vi "Untrained app.vi"() -> ()   [LabVIEW 2024]
panel:
  out "Instrument identificat":string
  in  "Classify":bool
  in  "Cale fisier audio":path
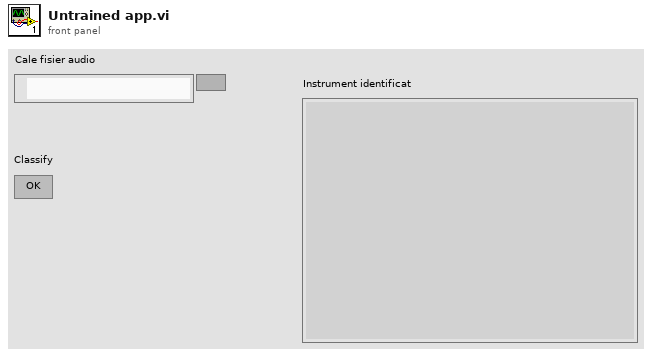
[diagram p1: front panel]
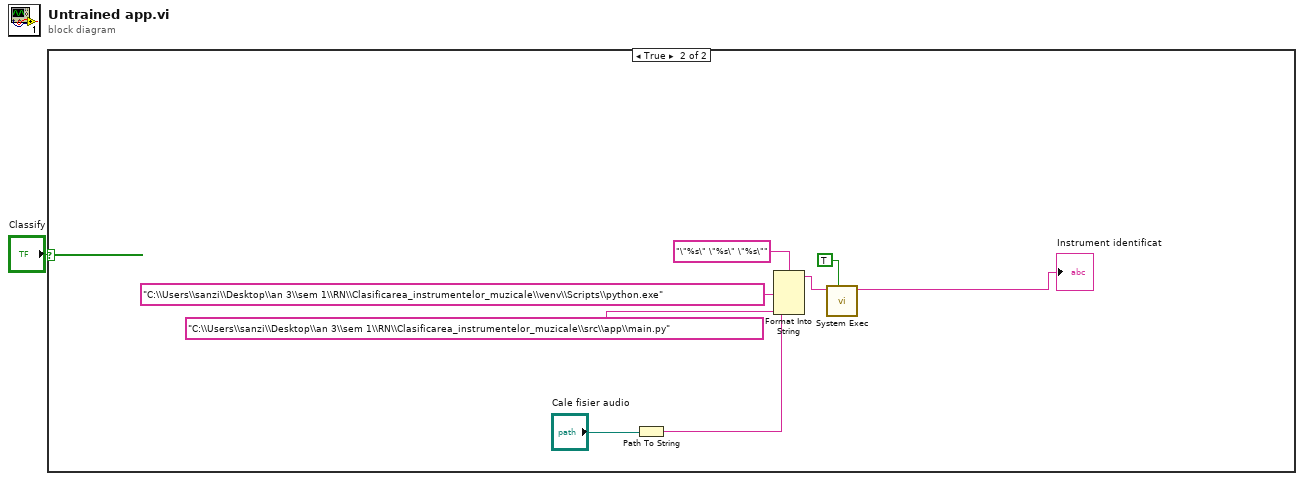
[diagram p0: block diagram]
diagram:
  n1 = case shown="True" "Classify" {
    frame False {
    }
    frame True {
      n2 = Path To String(path="Cale fisier audio") -> (string=w4:string)
      n3 = Format Into String(format string="\"%s\" \"%s\" \"%s\"", "C:\\Users\\sanzi\\Desktop\\an 3\\sem 1\\RN\\Clasificarea_instrumentelor_muzicale\\venv\\Scripts\\python.exe" ("input 1"), "C:\\Users\\sanzi\\Desktop\\an 3\\sem 1\\RN\\Clasificarea_instrumentelor_muzicale\\src\\app\\main.py" ("input 2"), w4) -> (resulting string=w3:string)  [unwired: 2 in, 1 out]
      n4 = call <vilib>:"System Exec.vi"("wait until completion? (T)"=TRUE, "command line"=w3) -> ("standard output"=→"Instrument identificat":string)  [unwired: 6 in, 3 out]
    }
  }
